vi "Get Schema Path.vi"(8 "error in (no error)":errorcluster) -> (0 "error out":errorcluster, 1 "Schema Path":string)   [LabVIEW 2013, in "Project Wizard.lvlib"]
uses:
  Project Wizard.lvlib
  <vilib>/Utility/sysdir.llb/System Directory Type.ctl
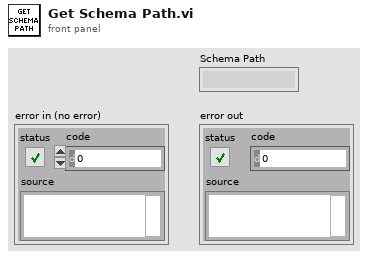
[diagram p1: front panel]
types:
  T1 = typedef "System Directory Type.ctl" = i32
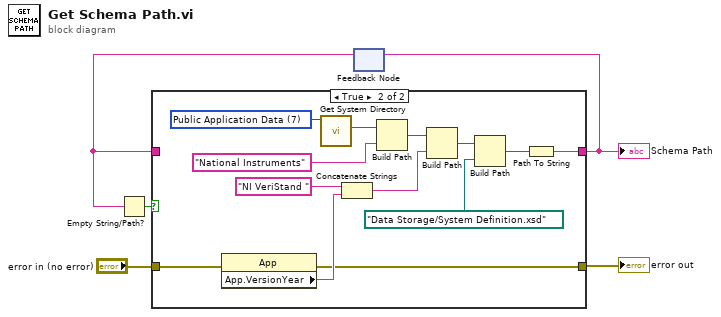
[diagram p0: block diagram]
diagram:
  n1 = feedback #1() -> (w1:string)  [unwired: 1 in]
  n2 = Empty String/Path?(string/path=w1) -> (empty?=w3:bool)
  n3 = case shown="True" w3 {
    tunnel: [w6 w10] -> w2
    tunnel: [w7 w9] -> w5
    tunnel: "error in (no error)" -> [w7 w8]
    tunnel: w1 -> [w6 _]
    frame False {
    }
    frame True {
      w20 = T1 7 items=["User Home"=0, "User Desktop"=1, "User Documents"=2, "User Application Data"=3, "User Preferences"=4, "User Temporary"=5, "Public Documents"=6, "Public Application Data"=7, "Public Preferences"=8, "Public Cache"=13, "System Core Libraries"=9, "System Installed Libraries"=10, "Application Files"=11, "Boot Volume Root"=12] ("system directory type")
      n4 = property class="App"(error in=w8) -> (error out=w9:errorcluster, "App.VersionYear"=w16:string)  [unwired: 1 in, 1 out]
      n5 = call <vilib>:"Get System Directory.vi"("system directory type"=w20) -> ("system directory"=w19:path)  [unwired: 10 in]
      n6 = Concatenate Strings("NI VeriStand " ("string"), w16) -> (w14:string)
      n7 = Build Path(base path=w19, name or relative path="National Instruments") -> (appended path=w15:path)
      n8 = Build Path(base path=w15, name or relative path=w14) -> (appended path=w13:path)
      n9 = Build Path(base path=w13, name or relative path=path "Data Storage/System Definition.xsd" ("appended path")) -> (appended path=w11:path)
      n10 = Path To String(path=w11) -> (string=w10:string)
    }
  }
  "error out" <- w5
  "Schema Path" <- w2
  n11 = feedback-in #1(w2) -> ()
